vi "List Installed Software Sets for Target.vi"() -> ()   [LabVIEW 2012]
uses:
  <vilib>/nisyscfg/Software Set 1.2.ctl
  <vilib>/nisyscfg/Software 1.2.ctl
  <vilib>/nisyscfg/Component Type.ctl
  <vilib>/nisyscfg/Get Available Sets.vi
  <vilib>/nisyscfg/Close (System).vi
  <vilib>/nisyscfg/nisyscfg.lvlib
panel:
  out "software sets":T1[](array[typedef]) {"information"."component type" items=["standard", "hidden", "system", "unknown", "startup"]; "items"."component type" items=["standard", "hidden", "system", "unknown", "startup"]; "add-ons"."component type" items=["standard", "hidden", "system", "unknown", "startup"]}
  out "error out":errorcluster
  in  "target (localhost)":refnum<k21>="localhost"
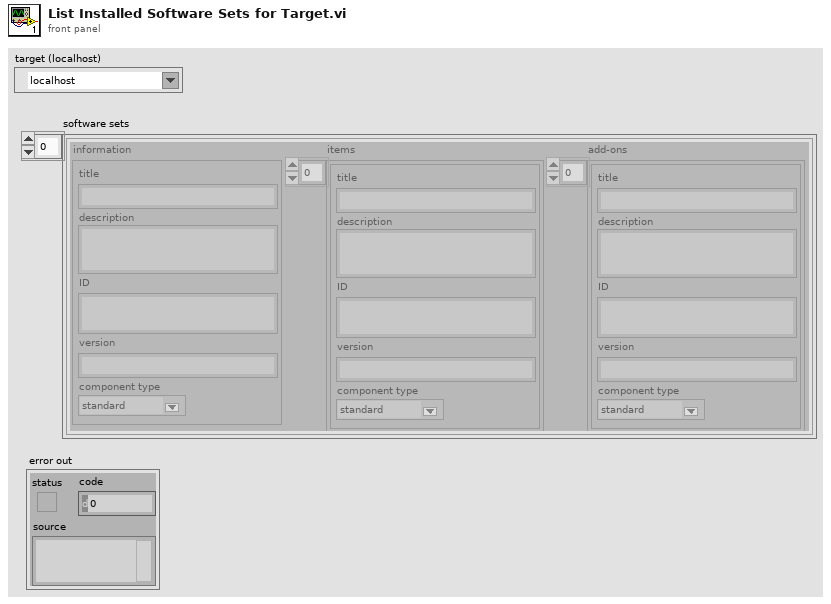
[diagram p1: front panel]
types:
  T1 = typedef "nisyscfg.lvlib/Software Set 1.2.ctl" = cluster{"information":T2, "items":T2[], "add-ons":T2[]}
  T2 = typedef "nisyscfg.lvlib/Software 1.2.ctl" = cluster{"title":string, "description":string, "ID":string, "version":string, "component type":T3}
  T3 = typedef "nisyscfg.lvlib/Component Type.ctl" = u32
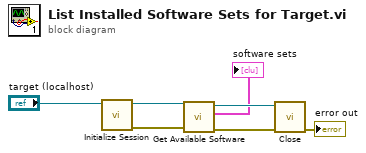
[diagram p0: block diagram]
diagram:
  n1 = call <vilib>:"Initialize Session.vi"("target (localhost)"="target (localhost)") -> ("error out"=w5:errorcluster, "session out"=w4:refnum<k21>)  [unwired: 9 in]
  n2 = call-poly <vilib>:"Get Available Software.vi"("error in (no error)"=w5, "session in"=w4) -> ("error out"=w3:errorcluster, "software sets"=→"software sets":T1[], "session out"=w7:refnum<k21>)  [unwired: 7 in]
  n3 = call-poly <vilib>:"Close.vi"("error in (no error)"=w3, "session in"=w7) -> ("error out"=→"error out":errorcluster)  [unwired: 9 in]
